vi "Final loop_with OPUS ver.vi"() -> ()   [LabVIEW 2015]
uses:
  <vilib>/DAQmx/read.llb/DAQmx Read (Analog 1D DBL 1Chan NSamp).vi
  <vilib>/DAQmx/create/channels.llb/DAQmx Create Channel (AI-Voltage-Basic).vi
  Global Variable.vi
  <vilib>/DAQmx/miscellaneous.llb/DAQmx Fill In Error Info.vi
panel:
  in  "Reset motor counts":bool
  out "Waveform Chart":cluster{dbl, "Actual Angle":dbl}(graph)={5.006659685432494, "Actual Angle"=5.006724697047278}
  out "Target Angle":dbl=5.006659685432494
  out "Actual Angle":dbl=5.006724697047278
  out "OPUS Voltage":dbl=-4.442503447248185 format="%0.4f"
  in  "Motor Speed":dbl(slide)=10.0 scale=0.0..10.0
  in  "reference angle":dbl=5.0
  in  "stop":bool
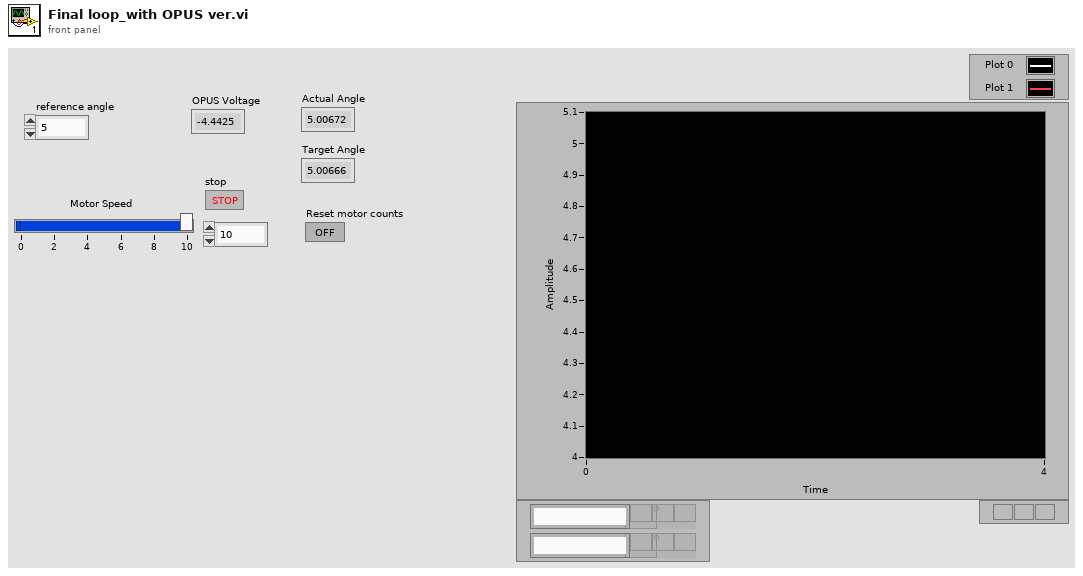
[diagram p1: front panel]
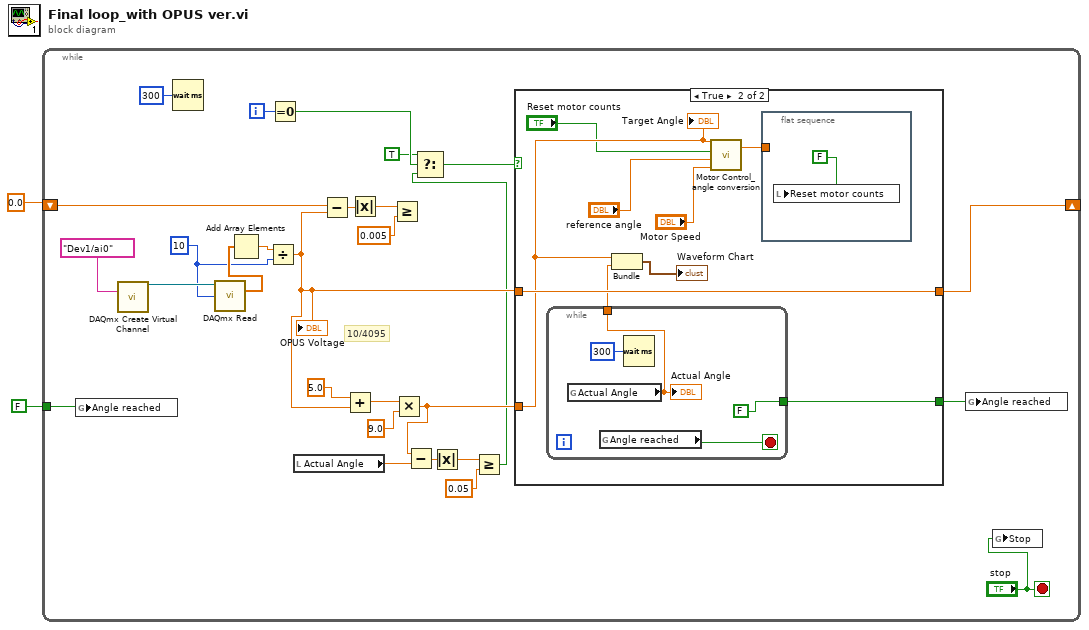
[diagram p0: block diagram]
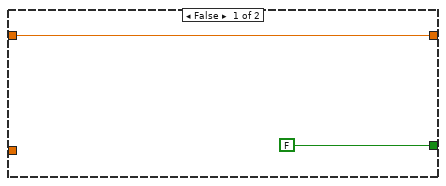
[diagram p2: hidden frame]
diagram:
  n1 = while {
    shift-right: [w25] -> _
    shift-left: 0.0 ("data") -> [w24]
    tunnel: FALSE -> [w15]
    i -> [w22]
    stop <- "stop" stop-if-true
    w17 = 10 ("number of samples per channel")
    # "10/4095"
    n2 = global write "Global Variable.vi" "Angle reached"(w15) -> ()
    n3 = call-poly <vilib>:"DAQmx Create Virtual Channel.vi"("physical channels"=tag "Dev1/ai0") -> ("task out"=w30:refnum<k21>)  [unwired: 13 in, 1 out]
    n4 = Wait (ms)(milliseconds to wait=u32 300) -> ()  [unwired: 1 out]
    n5 = call-poly <vilib>:"DAQmx Read.vi"("task/channels in"=w30, "number of samples per channel"=w17) -> ("data"=w19:dbl[])  [unwired: 11 in, 2 out]
    n6 = Add Array Elements(numeric array=w19) -> (sum=w18:dbl)
    n7 = Divide(x=w18, y=w17) -> (x/y=w11:dbl)
    "OPUS Voltage" <- w11
    n8 = Equal To 0?(x=w22) -> (x = 0?=w21:bool)
    n9 = local read "Actual Angle"() -> (w9:dbl)
    n10 = Subtract(x=w24, y=w11) -> (x-y=w28:dbl)
    n11 = Add(x=5.0, y=w11) -> (x+y=w12:dbl)
    n12 = Absolute Value(x=w28) -> (abs(x)=w27:dbl)
    n13 = Greater Or Equal?(x=w27, y=0.005) -> ()  [unwired: 1 out]
    n14 = Multiply(x=w12, y=9.0) -> (x*y=w10:dbl)
    n15 = Subtract(x=w10, y=w9) -> (x-y=w6:dbl)
    n16 = Absolute Value(x=w6) -> (abs(x)=w8:dbl)
    n17 = Greater Or Equal?(x=w8, y=0.05) -> (x >= y?=w5:bool)
    n18 = Select(t=TRUE, s=w21, f=w5) -> (s? t:f=w3:bool)
    n19 = case shown="True" w3 {
      tunnel: w11 -> [w32 w39]
      tunnel: [w32 w39] -> w25
      tunnel: [FALSE w38] -> w16
      tunnel: w10 -> [_ w37]
      frame False {
      }
      frame True {
        n20 = while {
          tunnel: [FALSE] -> w38
          tunnel: [w43] -> w36
          stop <- w45 stop-if-true
          n21 = global read "Global Variable.vi" "Actual Angle"() -> (w43:dbl)
          "Actual Angle" <- w43
          n22 = global read "Global Variable.vi" "Angle reached"() -> (w45:bool)
          n23 = Wait (ms)(milliseconds to wait=u32 300) -> ()  [unwired: 1 out]
        }
        n24 = Bundle(w37, "Actual Angle"=w36) -> (→"Waveform Chart":cluster{dbl, "Actual Angle":dbl})  [unwired: 1 in]
        n25 = call "Motor Control_ angle conversion.vi"("Motor Speed"="Motor Speed", "reference angle"="reference angle", "Reset motor counts"="Reset motor counts", "target angle"=w37) -> ("actual angle"=w33:dbl)  [unwired: 1 in]
        n26 = flat-sequence {
          tunnel: w33 -> [_]
          frame #0 {
            n27 = local write "Reset motor counts"(FALSE) -> ()
          }
        }
        "Target Angle" <- w37
      }
    }
    n28 = global write "Global Variable.vi" "Angle reached"(w16) -> ()
    n29 = global write "Global Variable.vi" "Stop"("stop") -> ()
  }
